vi "Connect to DAO.vi"(8 "error in (no error)":errorcluster, 9 "Object DAO JSON":refnum<class "Object DAO JSON.lvclass">, 10 "iObject":refnum<class "iObject.lvclass">) -> (0 "error out":errorcluster, 1 "Object DAO JSON out":refnum<class "Object DAO JSON.lvclass">)   [LabVIEW 2020, in "Object DAO Adapter.lvclass"]
uses:
  Object DAO Adapter.lvclass
  iObject/iObject.lvclass
  Object DAO JSON/Object DAO JSON.lvclass
  C:/Users/fflores/Desktop/DataBase - Copy - Copy/Object DAO/Object DAO.lvclass
  Object/Object.lvclass
  Object/Object.lvclass/Object.ctl
  Object DAO/Object DAO.lvclass/Object DAO.ctl
  Object DAO/Member Accessors/Get Object Information.vi
  Object/Member Accessors/Get String.vi
  Object/Member Accessors/Get Numeric.vi
  Object/Member Accessors/Get Boolean.vi
  Object DAO/Member Accessors/Set Object Information.vi
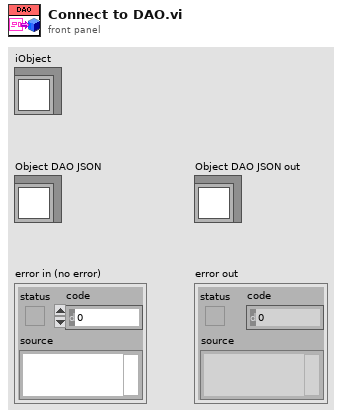
[diagram p1: front panel]
types:
  T1 = typedef "Object DAO.lvclass/Object Information.ctl" = cluster{"String":string, "Boolean":bool, "Numeric":dbl, "id":string}
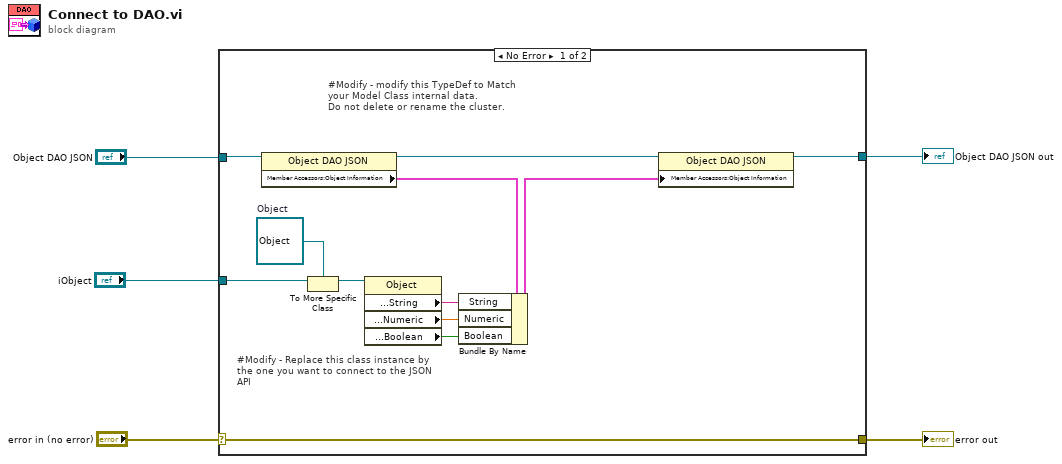
[diagram p0: block diagram]
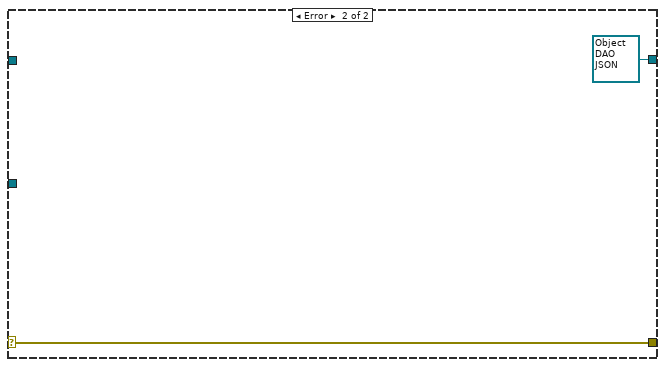
[diagram p2: hidden frame]
diagram:
  n1 = case shown="No Error" "error in (no error)" {
    selector: "error in (no error)" -> [w17 w19]
    tunnel: [w17 w19] -> w4
    tunnel: "iObject" -> [w15 _]
    tunnel: "Object DAO JSON" -> [w13 _]
    tunnel: [w6 refnum<class "Object DAO JSON.lvclass"> refnum ("Object DAO JSON")] -> w1
    frame No Error {
      w16 = refnum<class "Object.lvclass"> refnum  # Object
      # "#Modify - Replace this class instance by the one you want to connect to the JSON API"
      # "#Modify - modify this TypeDef to Match your Model Class internal data.\nDo not delete or rename the cluster."
      n2 = property class="Object DAO JSON"(reference=w13) -> (reference out=w12:refnum<class "Object DAO JSON.lvclass">, "Member Accessors:Object Information"=w11:T1)  [unwired: 1 in, 1 out]
      n3 = To More Specific Class(target class=w16, reference=w15) -> (specific class reference=w14:refnum<class "Object.lvclass">)  [unwired: 1 in, 1 out]
      n4 = property class="Object"(reference=w14) -> ("Member Accessors:String"=w9:string, "Member Accessors:Numeric"=w8:dbl, "Member Accessors:Boolean"=w7:bool)  [unwired: 1 in, 2 out]
      n5 = Bundle By Name(cluster=w11, "String"=w9, "Numeric"=w8, "Boolean"=w7) -> (w10:T1)
      n6 = property class="Object DAO JSON"(reference=w12, "Member Accessors:Object Information"=w10) -> (reference out=w6:refnum<class "Object DAO JSON.lvclass">)  [unwired: 1 in, 1 out]
    }
    frame Error {
    }
  }
  "error out" <- w4
  "Object DAO JSON out" <- w1
